vi "ReadSSF_DSF_两列DSF.vi"(11 "SF_PATH":string) -> (0 "DSF":cluster{"x":dbl, "y":dbl}[][](array[cluster]), 1 "因子棒号":string[](array[string]), 2 "SF_0K":bool, 3 "SSF":cluster{"x":dbl, "y":dbl}[][](array[cluster]), 5 "文件INFO":string)   [LabVIEW 2020]
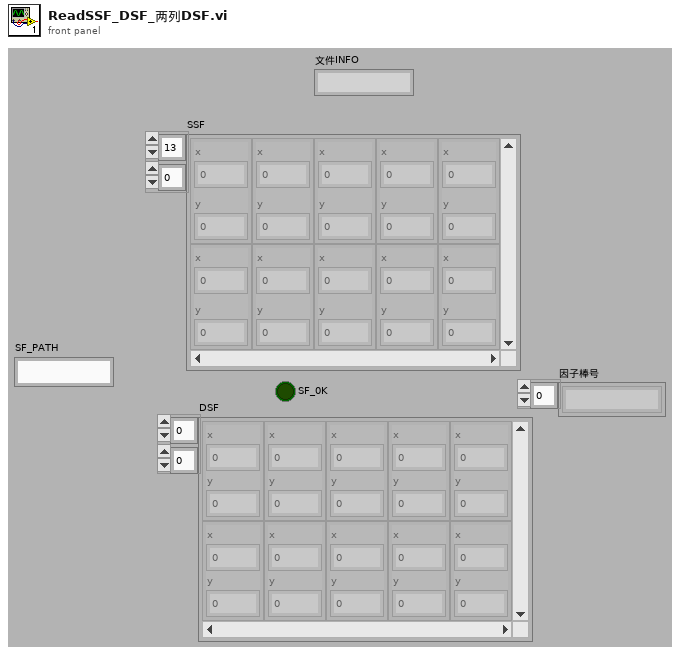
[diagram p1: front panel]
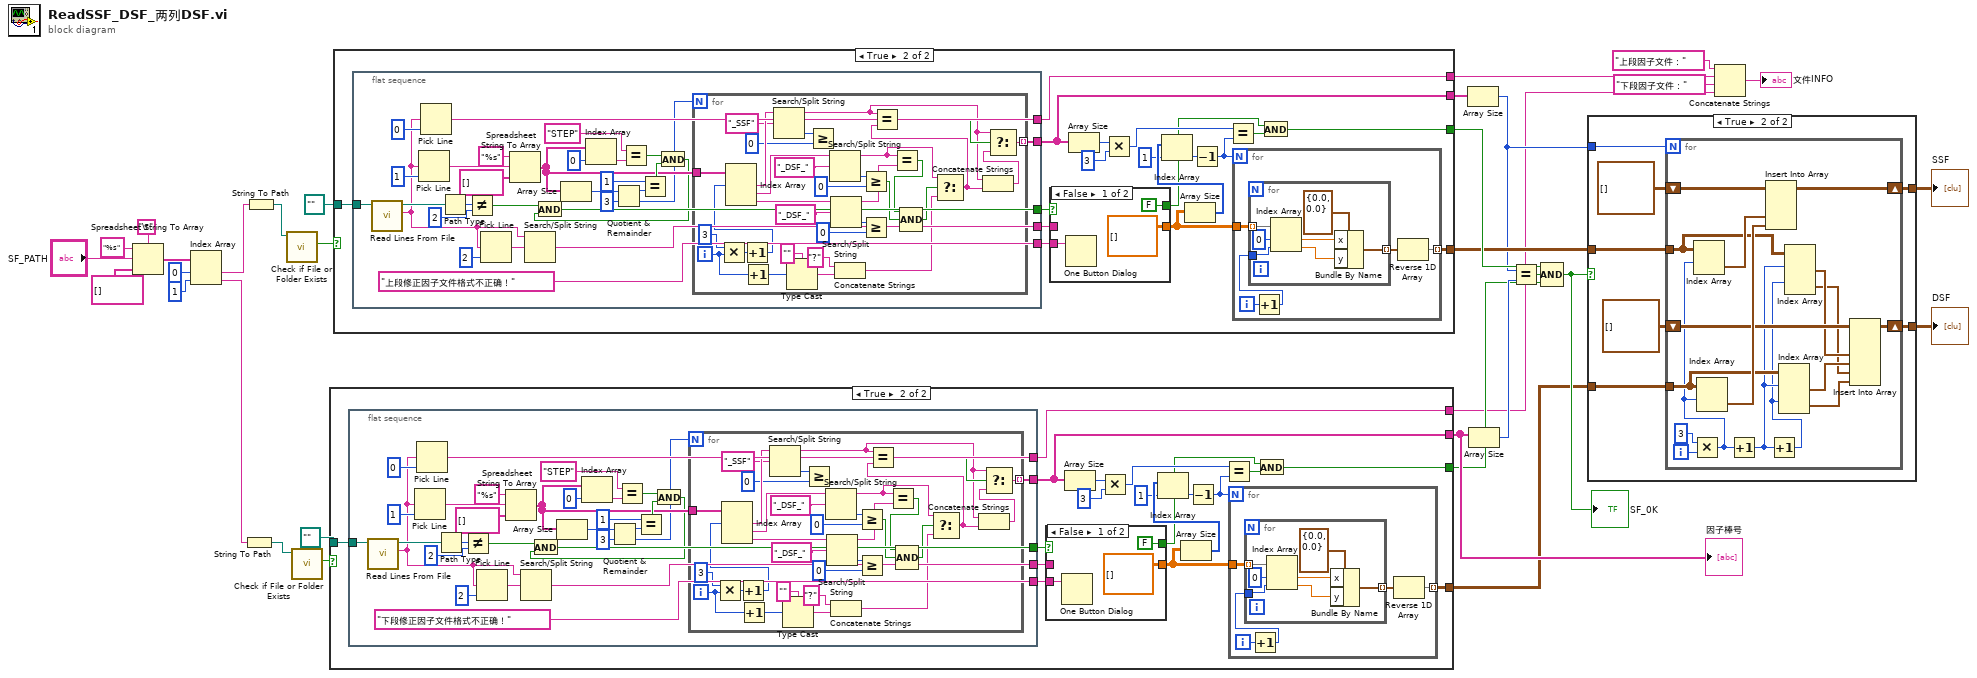
[diagram p0: block diagram]
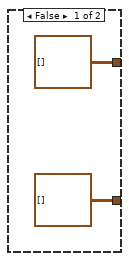
[diagram p2: hidden frame]
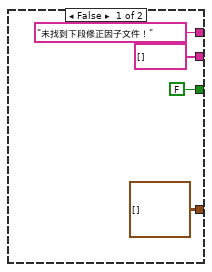
[diagram p3: hidden frame]
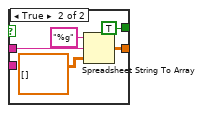
[diagram p4: hidden frame]
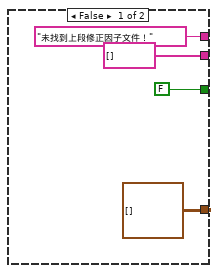
[diagram p5: hidden frame]
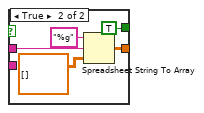
[diagram p6: hidden frame]
diagram:
  n1 = Spreadsheet String To Array(delimiter (Tab)="\t", format string="%s", spreadsheet string="SF_PATH", array type (2D Dbl)=string[] [] ("添加的数组")) -> (array=w25:string[])
  n2 = Index Array(array=w25, index #1=0 ("index"), index #2=1 ("index")) -> (element #1=w24:string, element #2=w23:string)
  n3 = String To Path(string=w23) -> (path=w20:path)
  n4 = String To Path(string=w24) -> (path=w32:path)
  n5 = call <vilib>:"Check if File or Folder Exists.vi"("path"=w32) -> ("file or folder exists?"=w31:bool)  [unwired: 8 in, 2 out]
  n6 = call <vilib>:"Check if File or Folder Exists.vi"("path"=w20) -> ("file or folder exists?"=w21:bool)  [unwired: 8 in, 2 out]
  n7 = case shown="True" w21 {
    tunnel: [cluster{"x":dbl, "y":dbl}[][] [] w50] -> w12
    tunnel: path "" -> [_ w51]
    tunnel: [FALSE ("file or folder exists?") w39] -> w15
    tunnel: ["未找到下段修正因子文件！" ("output string") w38] -> w1
    tunnel: [string[] [] w37] -> w18
    frame False {
    }
    frame True {
      n8 = flat-sequence {
        tunnel: [w92] -> w54
        tunnel: [w84] -> w53
        tunnel: ["下段修正因子文件格式不正确！" ("消息")] -> w52
        tunnel: w51 -> [w89]
        tunnel: [w83] -> w38
        tunnel: [w68] -> w37
        frame #0 {
          n9 = call <vilib>:"Read Lines From File.vi"("file path (dialog if empty)"=w89) -> ("new file path (Not A Path if cancelled)"=w91:path, "line string"=w85:string)  [unwired: 5 in, 2 out]
          n10 = Pick Line ("选行并添加至字符串")(multi-line string=w85, line index=1 ("行索引")) -> (output string=w81:string)  [unwired: 1 in]
          n11 = Pick Line ("选行并添加至字符串")(multi-line string=w85, line index=0 ("行索引")) -> (output string=w83:string)  [unwired: 1 in]
          n12 = Path Type(1:w91) -> (0:w95:i16)
          n13 = Not Equal?(x=w95, y=i16 2) -> (x != y?=w93:bool)
          n14 = Pick Line ("选行并添加至字符串")(multi-line string=w85, line index=2 ("行索引")) -> (output string=w86:string)  [unwired: 1 in]
          n15 = Spreadsheet String To Array ("电子表格字符串至数组转换")(format string="%s" ("format (%.3f)"), spreadsheet string=w81, array type (2D Dbl)=string[] [] ("添加的数组")) -> (array=w70:string[])  [unwired: 1 in]
          n16 = Search/Split String(string=w85, search string/char (-)=w86) -> (match + rest of string=w84:string)  [unwired: 1 in, 2 out]
          n17 = Array Size(array=w70) -> (size(s)=w76:i32)
          n18 = Index Array(array=w70, index=0 ("索引")) -> (element=w78:string)
          n19 = Quotient & Remainder(x=w76, y=3) -> (x-y*floor(x/y)=w74:i32, floor(x/y)=w69:i32)
          n20 = Equal?(x="STEP", y=w78) -> (x = y?=w71:bool)
          n21 = Equal?(x=1, y=w74) -> (x = y?=w72:bool)
          n22 = And(x=w71, y=w72) -> (x .and. y?=w67:bool)
          n23 = And(x=w93, y=w67) -> (x .and. y?=w92:bool)
          n24 = for {
            N: w69 -> [_]
            tunnel: w70 -> [w129]
            tunnel: [w108] -> w68 mode=indexing
            i -> [w110]
            n25 = Multiply(x=3, y=w110) -> (x*y=w127:i32)
            n26 = Increment(x=w127) -> (x+1=w126:i32)
            n27 = Index Array(array=w129, index #1=w126) -> (element #1=w125:string, element #2=w118:string, element #3=w114:string)  [unwired: 2 in]
            n28 = Increment(x=w110) -> (x+1=w109:i32)
            n29 = Search/Split String(string=w125, search string/char (-)="_SSF" ("搜索字符串/字符(-)")) -> (substring before match=w99:string, offset of match=w123:i32)  [unwired: 1 in, 1 out]
            n30 = Type Cast(type="" ("类型"), x=w109) -> (*(type *) &x=w107:string)
            n31 = Greater Or Equal?(x=w123, y=0) -> ()  [unwired: 1 out]
            n32 = Search/Split String(string=w118, search string/char (-)="_DSF_" ("搜索字符串/字符(-)")) -> (substring before match=w101:string, offset of match=w120:i32)  [unwired: 1 in, 1 out]
            n33 = Search/Split String(string=w114, search string/char (-)="_DSF_" ("搜索字符串/字符(-)")) -> (substring before match=w113:string, offset of match=w116:i32)  [unwired: 1 in, 1 out]
            n34 = Concatenate Strings("?" ("字符串"), w107) -> (w98:string)
            n35 = Greater Or Equal?(x=w120, y=0) -> (x >= y?=w104:bool)
            n36 = Greater Or Equal?(x=w116, y=0) -> (x >= y?=w105:bool)
            n37 = Equal?(x=w101, y=w113) -> (x = y?=w103:bool)
            n38 = Compound Arithmetic op=AND(w103, w104, w105) -> (w102:bool)
            n39 = Select(t=w101, s=w102, f=w98) -> (s? t:f=w97:string)
            n40 = Equal?(x=w99, y=w97) -> (x = y?=w112:bool)
            n41 = Concatenate Strings(w99, w97) -> (w100:string)
            n42 = Select(t=w99, s=w112, f=w100) -> (s? t:f=w108:string)
          }
        }
      }
      n43 = case shown="False" w54 {
        tunnel: w53 -> [_ w134]
        tunnel: [dbl[][] [] ("type (empty)") w135] -> w49
        tunnel: w52 -> [w131 _]
        tunnel: [FALSE ("file or folder exists?") TRUE ("file or folder exists?")] -> w40
        frame False {
          n44 = One Button Dialog(message=w131) -> ()  [unwired: 1 in, 1 out]
        }
        frame True {
          n45 = Spreadsheet String To Array ("电子表格字符串至数组转换")(format string="%g" ("format (%.3f)"), spreadsheet string=w134, array type (2D Dbl)=dbl[][] [] ("type (empty)")) -> (array=w135:dbl[][])  [unwired: 1 in]
        }
      }
      n46 = Array Size(array=w37) -> (size(s)=w45:i32)
      n47 = Multiply(x=w45, y=3) -> (x*y=w43:i32)
      n48 = Array Size(array=w49) -> (size(s)=w48:i32[])
      n49 = Index Array(array=w48, index=1 ("索引")) -> (element=w46:i32)
      n50 = Decrement(x=w46) -> (x-1=w42:i32)
      n51 = Equal?(x=w43, y=w42) -> (x = y?=w41:bool)
      n52 = for {
        N: w42 -> [_]
        tunnel: w49 -> [w58]
        tunnel: [w57] -> w50 mode=indexing
        i -> [w55]
        n53 = Increment(x=w55) -> (x+1=w56:i32)
        n54 = for {
          tunnel: w58 -> [w66] mode=indexing
          tunnel: [w64] -> w59 mode=indexing
          tunnel: w56 -> [w60]
          n55 = Index Array(array=w66, index #1=0 ("索引"), index #2=w60) -> (element #1=w62:dbl, element #2=w65:dbl)
          n56 = Bundle By Name(cluster=cluster{"x":dbl, "y":dbl} {"x"=0.0, "y"=0.0} ("输入簇"), "x"=w62, "y"=w65) -> (w64:cluster{"x":dbl, "y":dbl})
        }
        n57 = Reverse 1D Array(array=w59) -> (reversed array=w57:cluster{"x":dbl, "y":dbl}[])
      }
      n58 = And(x=w40, y=w41) -> (x .and. y?=w39:bool)
    }
  }
  "因子棒号" <- w18
  n59 = case shown="True" w31 {
    tunnel: [cluster{"x":dbl, "y":dbl}[][] [] w155] -> w13
    tunnel: path "" -> [_ w156]
    tunnel: [FALSE ("file or folder exists?") w144] -> w16
    tunnel: ["未找到上段修正因子文件！" ("output string") w143] -> w4
    tunnel: [string[] [] w142] -> w19
    frame False {
    }
    frame True {
      n60 = flat-sequence {
        tunnel: [w197] -> w159
        tunnel: [w189] -> w158
        tunnel: ["上段修正因子文件格式不正确！" ("消息")] -> w157
        tunnel: w156 -> [w194]
        tunnel: [w188] -> w143
        tunnel: [w173] -> w142
        frame #0 {
          n61 = call <vilib>:"Read Lines From File.vi"("file path (dialog if empty)"=w194) -> ("new file path (Not A Path if cancelled)"=w196:path, "line string"=w190:string)  [unwired: 5 in, 2 out]
          n62 = Pick Line ("选行并添加至字符串")(multi-line string=w190, line index=1 ("行索引")) -> (output string=w186:string)  [unwired: 1 in]
          n63 = Pick Line ("选行并添加至字符串")(multi-line string=w190, line index=0 ("行索引")) -> (output string=w188:string)  [unwired: 1 in]
          n64 = Path Type(1:w196) -> (0:w200:i16)
          n65 = Not Equal?(x=w200, y=i16 2) -> (x != y?=w198:bool)
          n66 = Pick Line ("选行并添加至字符串")(multi-line string=w190, line index=2 ("行索引")) -> (output string=w191:string)  [unwired: 1 in]
          n67 = Spreadsheet String To Array ("电子表格字符串至数组转换")(format string="%s" ("format (%.3f)"), spreadsheet string=w186, array type (2D Dbl)=string[] [] ("添加的数组")) -> (array=w175:string[])  [unwired: 1 in]
          n68 = Search/Split String(string=w190, search string/char (-)=w191) -> (match + rest of string=w189:string)  [unwired: 1 in, 2 out]
          n69 = Array Size(array=w175) -> (size(s)=w181:i32)
          n70 = Index Array(array=w175, index=0 ("索引")) -> (element=w183:string)
          n71 = Quotient & Remainder(x=w181, y=3) -> (x-y*floor(x/y)=w179:i32, floor(x/y)=w174:i32)
          n72 = Equal?(x="STEP", y=w183) -> (x = y?=w176:bool)
          n73 = Equal?(x=1, y=w179) -> (x = y?=w177:bool)
          n74 = And(x=w176, y=w177) -> (x .and. y?=w172:bool)
          n75 = And(x=w198, y=w172) -> (x .and. y?=w197:bool)
          n76 = for {
            N: w174 -> [_]
            tunnel: w175 -> [w234]
            tunnel: [w213] -> w173 mode=indexing
            i -> [w215]
            n77 = Multiply(x=3, y=w215) -> (x*y=w232:i32)
            n78 = Increment(x=w232) -> (x+1=w231:i32)
            n79 = Index Array(array=w234, index #1=w231) -> (element #1=w230:string, element #2=w223:string, element #3=w219:string)  [unwired: 2 in]
            n80 = Increment(x=w215) -> (x+1=w214:i32)
            n81 = Search/Split String(string=w230, search string/char (-)="_SSF" ("搜索字符串/字符(-)")) -> (substring before match=w204:string, offset of match=w228:i32)  [unwired: 1 in, 1 out]
            n82 = Type Cast(type="" ("类型"), x=w214) -> (*(type *) &x=w212:string)
            n83 = Greater Or Equal?(x=w228, y=0) -> ()  [unwired: 1 out]
            n84 = Search/Split String(string=w223, search string/char (-)="_DSF_" ("搜索字符串/字符(-)")) -> (substring before match=w206:string, offset of match=w225:i32)  [unwired: 1 in, 1 out]
            n85 = Search/Split String(string=w219, search string/char (-)="_DSF_" ("搜索字符串/字符(-)")) -> (substring before match=w218:string, offset of match=w221:i32)  [unwired: 1 in, 1 out]
            n86 = Concatenate Strings("?" ("字符串"), w212) -> (w203:string)
            n87 = Greater Or Equal?(x=w225, y=0) -> (x >= y?=w209:bool)
            n88 = Greater Or Equal?(x=w221, y=0) -> (x >= y?=w210:bool)
            n89 = Equal?(x=w206, y=w218) -> (x = y?=w208:bool)
            n90 = Compound Arithmetic op=AND(w208, w209, w210) -> (w207:bool)
            n91 = Select(t=w206, s=w207, f=w203) -> (s? t:f=w202:string)
            n92 = Equal?(x=w204, y=w202) -> (x = y?=w217:bool)
            n93 = Concatenate Strings(w204, w202) -> (w205:string)
            n94 = Select(t=w204, s=w217, f=w205) -> (s? t:f=w213:string)
          }
        }
      }
      n95 = case shown="False" w159 {
        tunnel: w158 -> [_ w239]
        tunnel: [dbl[][] [] ("type (empty)") w240] -> w154
        tunnel: w157 -> [w236 _]
        tunnel: [FALSE ("file or folder exists?") TRUE ("file or folder exists?")] -> w145
        frame False {
          n96 = One Button Dialog(message=w236) -> ()  [unwired: 1 in, 1 out]
        }
        frame True {
          n97 = Spreadsheet String To Array ("电子表格字符串至数组转换")(format string="%g" ("format (%.3f)"), spreadsheet string=w239, array type (2D Dbl)=dbl[][] [] ("type (empty)")) -> (array=w240:dbl[][])  [unwired: 1 in]
        }
      }
      n98 = Array Size(array=w142) -> (size(s)=w150:i32)
      n99 = Multiply(x=w150, y=3) -> (x*y=w148:i32)
      n100 = Array Size(array=w154) -> (size(s)=w153:i32[])
      n101 = Index Array(array=w153, index=1 ("索引")) -> (element=w151:i32)
      n102 = Decrement(x=w151) -> (x-1=w147:i32)
      n103 = Equal?(x=w148, y=w147) -> (x = y?=w146:bool)
      n104 = for {
        N: w147 -> [_]
        tunnel: w154 -> [w163]
        tunnel: [w162] -> w155 mode=indexing
        i -> [w160]
        n105 = Increment(x=w160) -> (x+1=w161:i32)
        n106 = for {
          tunnel: w163 -> [w171] mode=indexing
          tunnel: [w169] -> w164 mode=indexing
          tunnel: w161 -> [w165]
          n107 = Index Array(array=w171, index #1=0 ("索引"), index #2=w165) -> (element #1=w167:dbl, element #2=w170:dbl)
          n108 = Bundle By Name(cluster=cluster{"x":dbl, "y":dbl} {"x"=0.0, "y"=0.0} ("输入簇"), "x"=w167, "y"=w170) -> (w169:cluster{"x":dbl, "y":dbl})
        }
        n109 = Reverse 1D Array(array=w164) -> (reversed array=w162:cluster{"x":dbl, "y":dbl}[])
      }
      n110 = And(x=w145, y=w146) -> (x .and. y?=w144:bool)
    }
  }
  n111 = Array Size(array=w19) -> (size(s)=w11:i32)
  n112 = Array Size(array=w18) -> (size(s)=w17:i32)
  n113 = Equal?(x=w11, y=w17) -> (x = y?=w10:bool)
  n114 = Compound Arithmetic op=AND(w16, w10, w15) -> (w14:bool)
  "SF_0K" <- w14
  n115 = case shown="True" w14 {
    tunnel: w13 -> [_ w250]
    tunnel: w12 -> [_ w249]
    tunnel: w11 -> [_ w251]
    tunnel: [cluster{"x":dbl, "y":dbl}[][] [] w247] -> w9
    tunnel: [cluster{"x":dbl, "y":dbl}[][] [] w245] -> w6
    frame False {
    }
    frame True {
      n116 = for {
        N: w251 -> [_]
        tunnel: w250 -> [w260]
        tunnel: w249 -> [w259]
        shift-right: [w265] -> w247
        shift-left: cluster{"x":dbl, "y":dbl}[][] [] -> [w266]
        shift-right: [w261] -> w245
        shift-left: cluster{"x":dbl, "y":dbl}[][] [] -> [w262]
        i -> [w268]
        n117 = Multiply(x=3, y=w268) -> (x*y=w258:i32)
        n118 = Index Array(array=w260, index (row)=w258) -> (element=w264:cluster{"x":dbl, "y":dbl}[])  [unwired: 1 in]
        n119 = Index Array(array=w259, index (row)=w258) -> (element=w263:cluster{"x":dbl, "y":dbl}[])  [unwired: 1 in]
        n120 = Increment(x=w258) -> (x+1=w257:i32)
        n121 = Insert Into Array(array=w266, new element #1=w264, new element #2=w263) -> (w265:cluster{"x":dbl, "y":dbl}[][])  [unwired: 2 in]
        n122 = Increment(x=w257) -> (x+1=w256:i32)
        n123 = Index Array(array=w259, index (row) #1=w257, index (row) #2=w256) -> (element #1=w254:cluster{"x":dbl, "y":dbl}[], element #2=w252:cluster{"x":dbl, "y":dbl}[])  [unwired: 2 in]
        n124 = Index Array(array=w260, index (row) #1=w257, index (row) #2=w256) -> (element #1=w255:cluster{"x":dbl, "y":dbl}[], element #2=w253:cluster{"x":dbl, "y":dbl}[])  [unwired: 2 in]
        n125 = Insert Into Array(array=w262, new element #1=w255, new element #2=w254, new element #3=w253, new element #4=w252) -> (w261:cluster{"x":dbl, "y":dbl}[][])  [unwired: 2 in]
      }
    }
  }
  "SSF" <- w9
  "DSF" <- w6
  n126 = Concatenate Strings("上段因子文件：" ("字符串"), w4, "下段因子文件：" ("字符串"), w1) -> (→"文件INFO":string)
